vi "R30_1-FPGA.vi"() -> ()   [LabVIEW 2016]
uses:
  control vi/controls/Glassman Control.ctl
  control vi/controls/Faraday Cup Readback.ctl
  control vi/controls/Aperture Readback.ctl
  <vilib>/LabVIEW Targets/FPGA/cRIO/shared/nicrio_ModuleControls/nicrio_cRIO-9871_BaudRateEnum.ctl
  <vilib>/LabVIEW Targets/FPGA/cRIO/shared/nicrio_ModuleControls/nicrio_cRIO-9871_ParityEnum.ctl
  <vilib>/LabVIEW Targets/FPGA/cRIO/shared/nicrio_ModuleControls/nicrio_cRIO-9871_StopBitsEnum.ctl
  <vilib>/LabVIEW Targets/FPGA/cRIO/shared/nicrio_ModuleControls/nicrio_cRIO-9871_DataBitsEnum.ctl
  <vilib>/Platform/TimedLoop/XDataNode/timing_clust.ctl
  <vilib>/Platform/TimedLoop/XDataNode/nitl_modes.ctl
  <vilib>/Platform/TimedLoop/XDataNode/wakeup.ctl
  <vilib>/rvi/FXPMathLib/basic elements/FxpIntAccumulator/subVIs/nifxpmath_IntAccumulator_SimConfig.ctl
  <vilib>/rvi/Emulation/niFpgaGetClockAttributes.vi
  <vilib>/rvi/Emulation/niFpgaSctlEmulationGetInTimedLoop.vi
  <vilib>/rvi/Emulation/niFpgaEmulationReportErrorSimple.vi
  <vilib>/rvi/eio/common/nirviEmuTemplateMethod_errors.vi
  <vilib>/rvi/Analysis/common/codeGenErrors/XNode/niFpgaXNodeCodeGenErrorHandle.vi
  <vilib>/rvi/Emulation/niFpgaCriticalErrorInLSC.vi
  <vilib>/rvi/FXPMathLib/basic elements/FxpIntAccumulator/simVIs/DllFxpIntAccumulator_sub.vi
  <vilib>/rvi/eio/common/nirviEmuTemplatePropertySet_errors.vi
  <vilib>/eio/EIONode/EIONode.xnode
  <vilib>/rvi/Analysis/measure/dc-rms/XNode/niFpgaDC-RMS.xnode
  <vilib>/Platform/TimedLoop/XDataNode/XDataNode.xnode
  <vilib>/rvi/FXPMathLib/basic elements/FxpIntAccumulator/XNode/nifxpmath_IntAccumulator.xnode
  <vilib>/rvi/FXPMathLib/FxpMul/XNode/nifxpmath_Multiplier.xnode
  <vilib>/eio/EIOPropertyNode/EIOPropertyNode.xnode
  <vilib>/eio/EIOMethodNode/EIOMethodNode.xnode
  <vilib>/Platform/TimedLoop/XDataNode/XDNodeRunTimeDep.lvlib
  <vilib>/rvi/FXPMathLib/sim/FxpSim.dll
  <vilib>/rvi/eio/common/nirviEmuTemplatePropertyGet_errors.vi
  <vilib>/rvi/eio/common/nirviEmuTemplatePropertyGet_noerrors.vi
  <vilib>/rvi/eio/common/nirviEmuTemplatePropertySet_noerrors.vi
panel:
  out "ESA V read":fxp<+/-,26,5>
  out "ESA I read":fxp<+/-,26,5>
  out "X+ Steerer V read":fxp<+/-,26,5>
  out "X+ Steerer I read":fxp<+/-,26,5>
  out "X- Steerer V read":fxp<+/-,26,5>
  out "X- Steerer I read":fxp<+/-,26,5>
  out "Y+ Steerer V read":fxp<+/-,26,5>
  out "Y+ Steerer I read":fxp<+/-,26,5>
  out "Y- Steerer V read":fxp<+/-,26,5>
  out "Y- Steerer I read":fxp<+/-,26,5>
  out "Mag Steerer V read":fxp<+/-,26,5>
  out "Mag Steerer I read":fxp<+/-,26,5>
  out "HV readback loop error":errorcluster
  out "Quad B I read":fxp<+/-,26,5>
  out "Quad A I read":fxp<+/-,26,5>
  in  "RT error":bool
  out "Switch Magnet Aperture Position":T1
  out "Detector Aperture Position":T1
  out "Detector FC Position":T2
  out "Switch Magnet FC Position":T2
  out "Actuator loop error":errorcluster
  in  "Y- Steerer V set":T3
  in  "Y+ Steerer V set":T3
  in  "X- Steerer V set":T3
  in  "X+ Steerer V set":T3
  in  "Quad B set":fxp<+/-,20,5>
  in  "Quad A set":fxp<+/-,20,5>
  in  "ESA Voltage set":fxp<+/-,20,5>
  out "HV control loop error":errorcluster
  out "Cryo Readback error":errorcluster
  out "Vacuum Gauge 1 error":errorcluster
  out "Vacuum Gauge 2 error":errorcluster
  out "Vacuum Gauge 3 error":errorcluster
  out "Switch Image Ion Gauge 1":u8[](array[numeric])
  out "Switch Image Convectron 1":u8[](array[numeric])
  out "Time since repurge":u8[](array[numeric])
  out "1st stage temp":u8[](array[numeric])
  out "2nd stage temp":u8[](array[numeric])
  out "Cryo On-time":u8[](array[numeric])
  out "Cryo Status":u8[](array[numeric])
  out "R30 ESA Convectron  1":u8[](array[numeric])
  out "R30 ESA Ion gauge 1":u8[](array[numeric])
  out "R30 Detector Convectron  1":u8[](array[numeric])
  out "R30 Detector Ion gauge 1":u8[](array[numeric])
  in  "Mag Steerer I-program":fxp<+/-,20,5> format="%.17g"
  in  "Switch magnet Aperture Actuator":bool
  in  "Detector Aperture Actuator":bool
  in  "Detector FC Actuator":bool
  in  "Switch magnet FC Actuator":bool
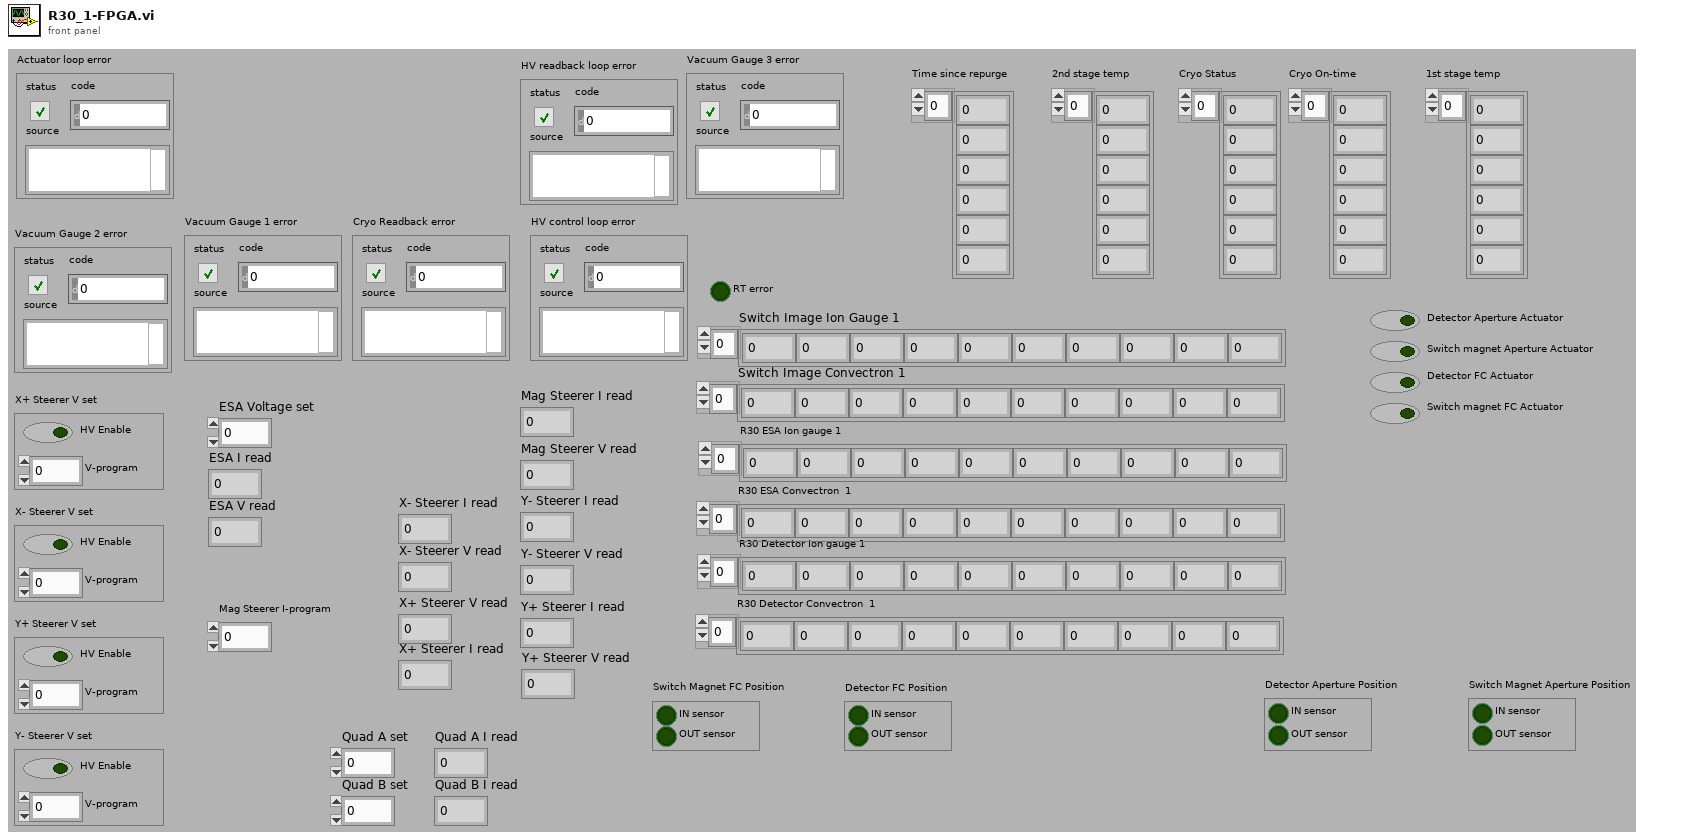
[diagram p1: front panel]
types:
  T1 = typedef "Aperture Readback.ctl" = cluster{"IN sensor":bool, "OUT sensor":bool}
  T2 = typedef "Faraday Cup Readback.ctl" = cluster{"IN sensor":bool, "OUT sensor":bool}
  T3 = typedef "Glassman Control.ctl" = cluster{"V-program":fxp<+/-,16,5>, "HV Enable":bool}
  T4 = typedef "nicrio_cRIO-9871_StopBitsEnum.ctl" = enum8{"1", "1.5", "2"}
  T5 = typedef "nicrio_cRIO-9871_ParityEnum.ctl" = enum8{"None", "Odd", "Even", "Mark", "Space"}
  T6 = typedef "nicrio_cRIO-9871_DataBitsEnum.ctl" = enum8{"5", "6", "7", "8"}
  T7 = typedef "nicrio_cRIO-9871_BaudRateEnum.ctl" = enum16{"75 bps", "110 bps", "134 bps", "150 bps", "300 bps", "600 bps", "1200 bps", "1800 bps", "2400 bps", "4800 bps", "7200 bps", "9600 bps", "14.4 kbps", "19.2 kbps", "28.8 kbps", "38.4 kbps", "57.6 kbps", "115.2 kbps", "230.4 kbps", "460.8 kbps", "921.6 kbps"}
  T8 = typedef "XDNodeRunTimeDep.lvlib/timing_clust.ctl" = cluster{"Expected End [f-1]":u64, "Actual End [f-1]":u64, "Finished Late? [f-1]":bool, "Expected End [i-1]":u64, "Actual End [i-1]":u64, "Finished Late? [i-1]":bool, "Expected Start [i]":u64, "Actual Start [i]":u64, "Expected Start [f]":u64, "Actual Start [f]":u64, "Source Name":string, "Structure Name":string, "Period":i64, "Deadline":i64, "Offset":i64, "Start":i64, "Priority":i32, "Timeout":i32, "Mode":T9, "Wakeup Reason":T10, "Error":errorcluster, "Source Type":string, "Secondary Source Type":string, "Global End Time":u64, "Global Start Time":u64, "Frame Duration":u64, "Iteration Duration":u64, "Assigned CPU":i32, "I/O Scan Engine Mode":u32}
  T9 = typedef "XDNodeRunTimeDep.lvlib/nitl_modes.ctl" = enum32{"No Change", "Process missed periods, maintain original phase", "Discard missed periods, maintain original phase", "Process missed periods, ignore original phase", "Discard missed periods, ignore original phase"}
  T10 = typedef "XDNodeRunTimeDep.lvlib/wakeup.ctl" = enum32{"Normal", "Aborted", "Asynchronous wakeup", "Timing source error", "Timed loop error", "Timeout"}
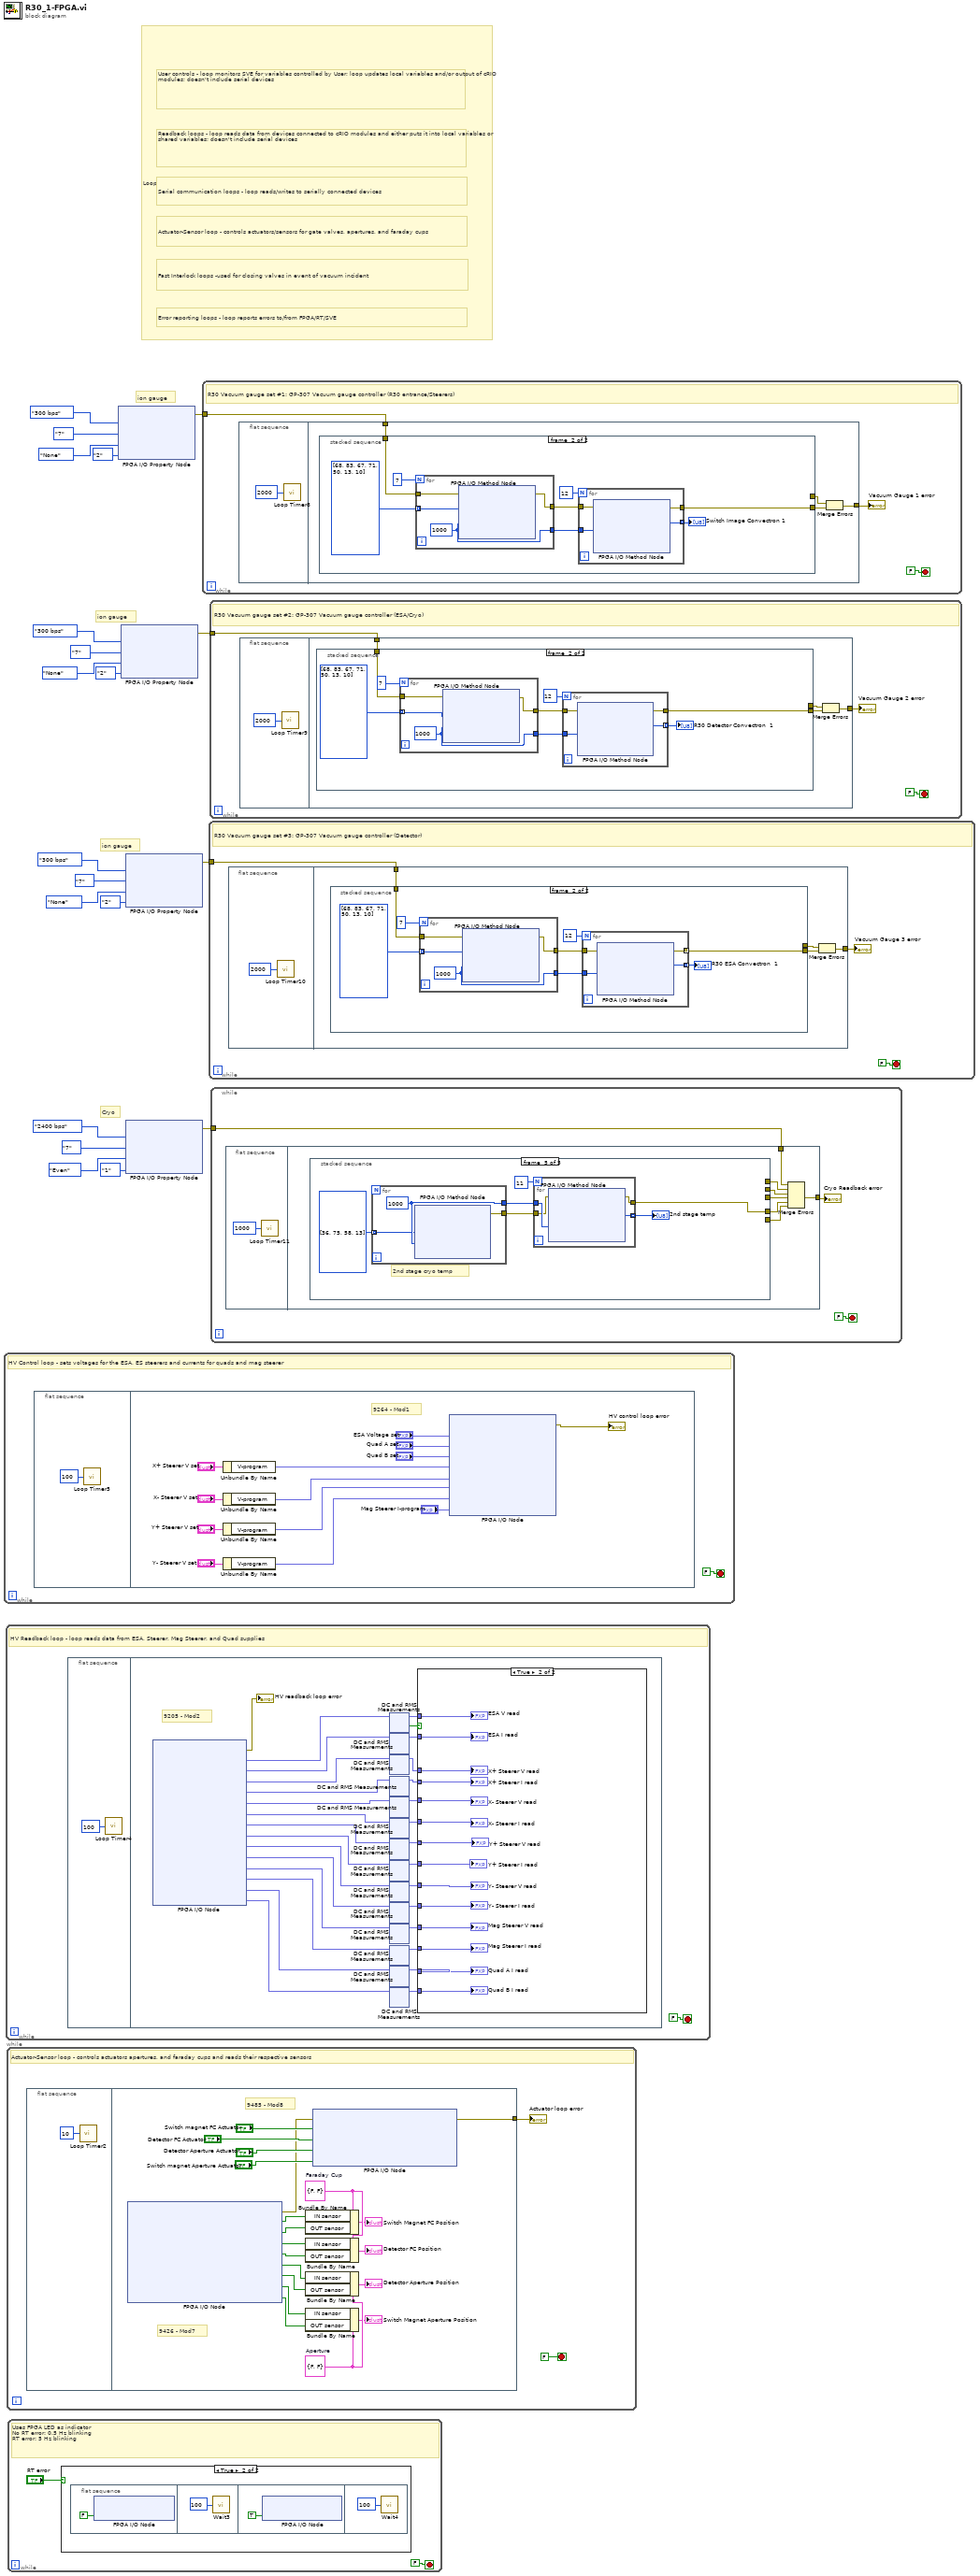
[diagram p0: block diagram]
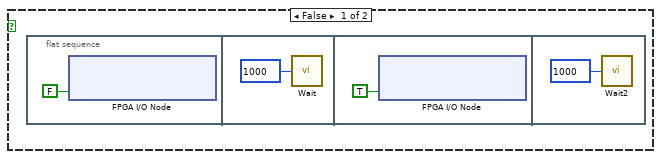
[diagram p2: hidden frame]
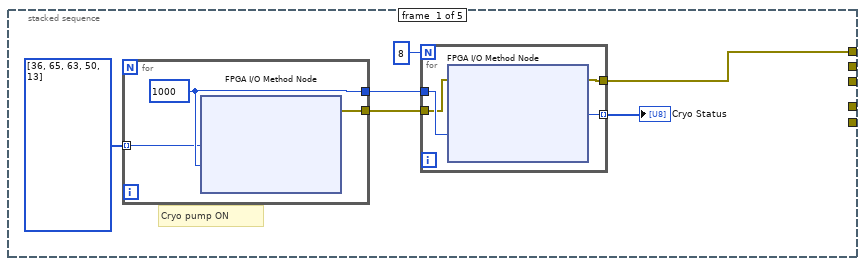
[diagram p3: hidden frame]
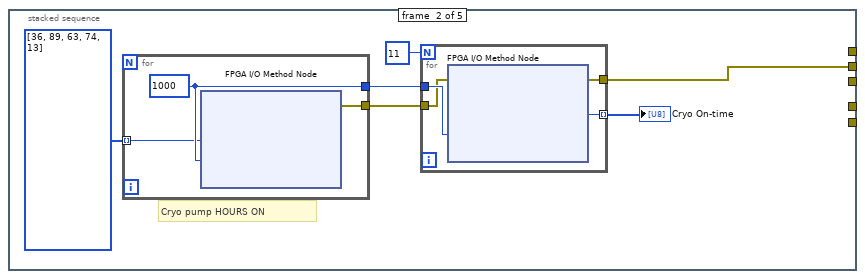
[diagram p4: hidden frame]
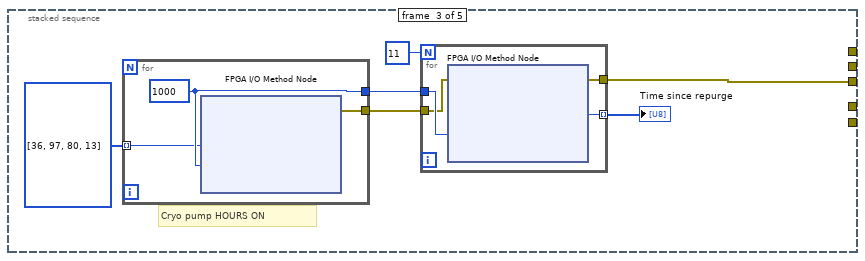
[diagram p5: hidden frame]
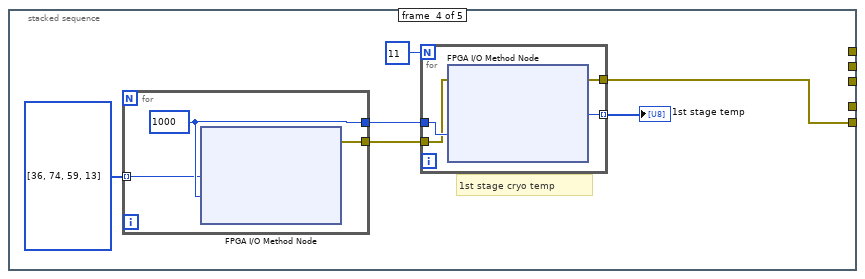
[diagram p6: hidden frame]
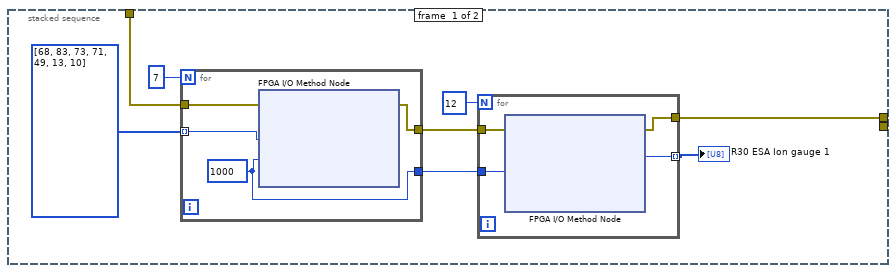
[diagram p7: hidden frame]
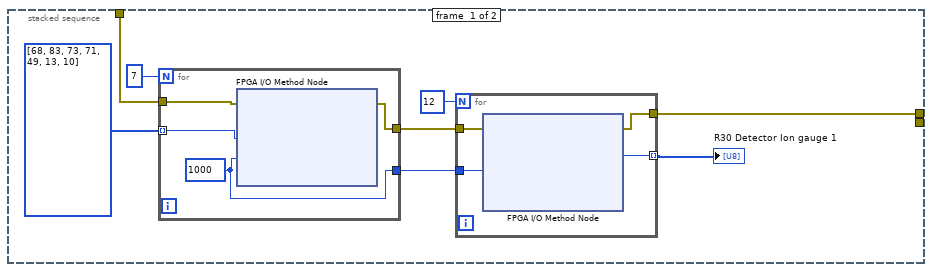
[diagram p8: hidden frame]
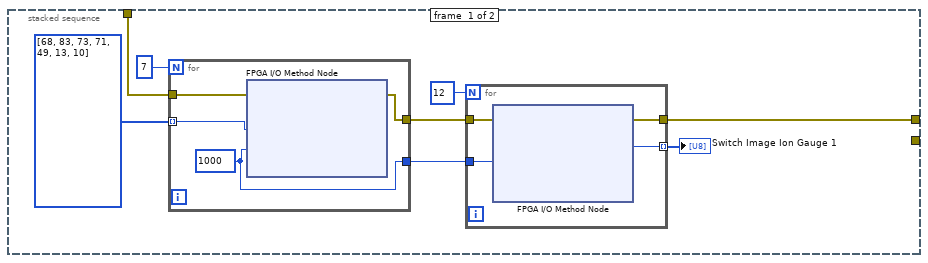
[diagram p9: hidden frame]
diagram:
  # "Actuator-Sensor loop - controls actuators/sensors for gate valves, apertures, and faraday cups"
  # "Fast Interlock loops -used for closing valves in event of vacuum incident"
  # "Error reporting loops - loop reports errors to/from FPGA/RT/SVE"
  # "Serial communication loops - loop reads/writes to serially connected devices"
  # "Readback loops - loop reads data from devices connected to cRIO modules and either puts it into local variables or shared variables; doesn't include serial devices"
  # "User controls - loop monitors SVE for variables controlled by User; loop updates local variables and/or output of cRIO modules; doesn't include serial devices"
  # "Loop legend - loops are color coded by responsibility"
  # "Cryo"
  # "ion gauge"
  # "ion gauge"
  # "ion gauge"
  n1 = while {
    stop <- FALSE stop-if-true
    # "HV Control loop - sets voltages for the ESA, ES steerers and currents for quads and mag steerer"
    n2 = flat-sequence {
      frame #0 {
        n3 = call "Loop Timer5"("Count(mSec)"=u32 100) -> ()  [unwired: 1 out]
      }
      frame #1 {
        # "9264 - Mod1"
        n4 = Unbundle By Name("X+ Steerer V set") -> ("V-program"=w26:fxp<+/-,16,5>)
        n5 = Unbundle By Name("X- Steerer V set") -> ("V-program"=w25:fxp<+/-,16,5>)
        n6 = Unbundle By Name("Y+ Steerer V set") -> ("V-program"=w24:fxp<+/-,16,5>)
        n7 = Unbundle By Name("Y- Steerer V set") -> ("V-program"=w23:fxp<+/-,16,5>)
        n8 = xnode "FPGA I/O Node"("ESA Voltage set"="ESA Voltage set", "Quad A set"="Quad A set", "Quad B set"="Quad B set", "X+ Steerer V set"=w26, "X- Steerer V set"=w25, "Y+ Steerer V set"=w24, "Y- Steerer V set"=w23, "Mag Steerer I-program"="Mag Steerer I-program") -> ("error out"=→"HV control loop error":errorcluster)  [unwired: 9 in, 8 out]
      }
    }
  }
  n9 = while {
    stop <- FALSE stop-if-true
    # "HV Readback loop - loop reads data from ESA, Steerer, Mag Steerer, and Quad supplies"
    n10 = flat-sequence {
      frame #0 {
        n11 = call "Loop Timer4"("Count(mSec)"=u32 100 ("Count(Ticks)")) -> ()  [unwired: 1 out]
      }
      frame #1 {
        # "9205 - Mod2"
        n12 = xnode "FPGA I/O Node"() -> ("error out"=→"HV readback loop error":errorcluster, "ESA V read"=w58:fxp<+/-,26,5>, "ESA I read"=w57:fxp<+/-,26,5>, "X+ Steerer V read"=w56:fxp<+/-,26,5>, "X+ Steerer I read"=w55:fxp<+/-,26,5>, "X- Steerer V read"=w54:fxp<+/-,26,5>, "X- Steerer I read"=w53:fxp<+/-,26,5>, "Y+ Steerer V read"=w52:fxp<+/-,26,5>, "Y+ Steerer I read"=w51:fxp<+/-,26,5>, "Y- Steerer V read"=w46:fxp<+/-,26,5>, "Y- Steerer I read"=w45:fxp<+/-,26,5>, "Mag Steerer V read"=w44:fxp<+/-,26,5>, "Mag Steerer I read"=w43:fxp<+/-,26,5>, "Quad A I read"=w42:fxp<+/-,26,5>, "Quad B I read"=w41:fxp<+/-,26,5>)  [unwired: 15 in, 14 out]
        n13 = xnode "DC and RMS Measurements"("input data"=w58) -> ("DC"=w66:fxp<+/-,26,5>, "output valid"=w67:bool)  [unwired: 1 in]
        n14 = xnode "DC and RMS Measurements"("input data"=w57) -> ("DC"=w65:fxp<+/-,26,5>)  [unwired: 1 in, 1 out]
        n15 = xnode "DC and RMS Measurements"("input data"=w56) -> ("DC"=w64:fxp<+/-,26,5>)  [unwired: 1 in, 1 out]
        n16 = xnode "DC and RMS Measurements"("input data"=w55) -> ("DC"=w63:fxp<+/-,26,5>)  [unwired: 1 in, 1 out]
        n17 = xnode "DC and RMS Measurements"("input data"=w54) -> ("DC"=w62:fxp<+/-,26,5>)  [unwired: 1 in, 1 out]
        n18 = xnode "DC and RMS Measurements"("input data"=w53) -> ("DC"=w61:fxp<+/-,26,5>)  [unwired: 1 in, 1 out]
        n19 = xnode "DC and RMS Measurements"("input data"=w52) -> ("DC"=w60:fxp<+/-,26,5>)  [unwired: 1 in, 1 out]
        n20 = xnode "DC and RMS Measurements"("input data"=w51) -> ("DC"=w59:fxp<+/-,26,5>)  [unwired: 1 in, 1 out]
        n21 = xnode "DC and RMS Measurements"("input data"=w46) -> ("DC"=w50:fxp<+/-,26,5>)  [unwired: 1 in, 1 out]
        n22 = xnode "DC and RMS Measurements"("input data"=w45) -> ("DC"=w49:fxp<+/-,26,5>)  [unwired: 1 in, 1 out]
        n23 = xnode "DC and RMS Measurements"("input data"=w44) -> ("DC"=w48:fxp<+/-,26,5>)  [unwired: 1 in, 1 out]
        n24 = xnode "DC and RMS Measurements"("input data"=w43) -> ("DC"=w47:fxp<+/-,26,5>)  [unwired: 1 in, 1 out]
        n25 = xnode "DC and RMS Measurements"("input data"=w42) -> ("DC"=w40:fxp<+/-,26,5>)  [unwired: 1 in, 1 out]
        n26 = xnode "DC and RMS Measurements"("input data"=w41) -> ("DC"=w39:fxp<+/-,26,5>)  [unwired: 1 in, 1 out]
        n27 = case shown="True" w67 {
          tunnel: w66 -> [_ w721]
          tunnel: w65 -> [_ w720]
          tunnel: w64 -> [_ w719]
          tunnel: w63 -> [_ w718]
          tunnel: w62 -> [_ w717]
          tunnel: w61 -> [_ w716]
          tunnel: w60 -> [_ w715]
          tunnel: w59 -> [_ w714]
          tunnel: w50 -> [_ w713]
          tunnel: w49 -> [_ w712]
          tunnel: w48 -> [_ w711]
          tunnel: w47 -> [_ w710]
          tunnel: w40 -> [_ w709]
          tunnel: w39 -> [_ w708]
          frame False {
          }
          frame True {
            "Quad A I read" <- w709
            "Quad B I read" <- w708
            "Mag Steerer I read" <- w710
            "Mag Steerer V read" <- w711
            "Y- Steerer I read" <- w712
            "Y- Steerer V read" <- w713
            "Y+ Steerer I read" <- w714
            "Y+ Steerer V read" <- w715
            "X- Steerer I read" <- w716
            "X- Steerer V read" <- w717
            "X+ Steerer I read" <- w718
            "X+ Steerer V read" <- w719
            "ESA I read" <- w720
            "ESA V read" <- w721
          }
        }
      }
    }
  }
  n28 = while {
    stop <- FALSE stop-if-true
    # "Actuator-Sensor loop - controls actuators apertures, and faraday cups and reads their respective sensors"
    n29 = flat-sequence {
      tunnel: [w1222] -> w1202
      frame #0 {
        n30 = call "Loop Timer2"("Count(uSec)"=u32 10) -> ()  [unwired: 1 out]
      }
      frame #1 {
        w1211 = T1 {"IN sensor"=FALSE, "OUT sensor"=FALSE}  # Aperture
        w1214 = T2 {"IN sensor"=FALSE, "OUT sensor"=FALSE}  # Faraday Cup
        # "9485 - Mod8"
        # "9426 - Mod7"
        n31 = xnode "FPGA I/O Node"() -> ("error out"=w1219:errorcluster, "Switch Magnet FC IN sensor"=w1218:bool, "Switch Magnet FC OUT sensor"=w1217:bool, "Detector FC IN sensor"=w1216:bool, "Detector FC OUT sensor"=w1215:bool, "Detector Aperture IN sensor"=w1207:bool, "Detector Aperture OUT sensor"=w1208:bool, "Switch Magnet Aperture IN sensor"=w1209:bool, "Switch Magnet Aperture OUT sensor"=w1210:bool)  [unwired: 9 in, 8 out]
        n32 = Bundle By Name(cluster=w1214, "IN sensor"=w1218, "OUT sensor"=w1217) -> (→"Switch Magnet FC Position":T2)
        n33 = Bundle By Name(cluster=w1214, "IN sensor"=w1216, "OUT sensor"=w1215) -> (→"Detector FC Position":T2)
        n34 = Bundle By Name(cluster=w1211, "IN sensor"=w1207, "OUT sensor"=w1208) -> (→"Detector Aperture Position":T1)
        n35 = Bundle By Name(cluster=w1211, "IN sensor"=w1209, "OUT sensor"=w1210) -> (→"Switch Magnet Aperture Position":T1)
        n36 = xnode "FPGA I/O Node"("error in"=w1219, "Switch Magnet FC Actuator"="Switch magnet FC Actuator", "Detector FC Actuator"="Detector FC Actuator", "Detector Aperture Actuator"="Detector Aperture Actuator", "Switch Magnet Aperture Actuator"="Switch magnet Aperture Actuator") -> ("error out"=w1222:errorcluster)  [unwired: 4 in, 4 out]
      }
    }
    "Actuator loop error" <- w1202
  }
  n37 = while {
    stop <- FALSE stop-if-true
    # "Uses FPGA LED as indicator\nNo RT error: 0.5 Hz blinking\nRT error: 5 Hz blinking"
    n38 = case shown="True" "RT error" {
      frame False {
        n39 = flat-sequence {
          frame #0 {
            n40 = xnode "FPGA I/O Node"("USER FPGA LED"=FALSE ("FPGA LED")) -> ()  [unwired: 1 in, 1 out]
          }
          frame #1 {
            n41 = call "Wait"("Count(mSec)"=u16 1000) -> ()  [unwired: 1 out]
          }
          frame #2 {
            n42 = xnode "FPGA I/O Node"("USER FPGA LED"=TRUE ("FPGA LED")) -> ()  [unwired: 1 in, 1 out]
          }
          frame #3 {
            n43 = call "Wait2"("Count(mSec)"=u16 1000) -> ()  [unwired: 1 out]
          }
        }
      }
      frame True {
        n44 = flat-sequence {
          frame #0 {
            n45 = xnode "FPGA I/O Node"("USER FPGA LED"=FALSE ("FPGA LED")) -> ()  [unwired: 1 in, 1 out]
          }
          frame #1 {
            n46 = call "Wait3"("Count(mSec)"=u16 100) -> ()  [unwired: 1 out]
          }
          frame #2 {
            n47 = xnode "FPGA I/O Node"("USER FPGA LED"=TRUE ("FPGA LED")) -> ()  [unwired: 1 in, 1 out]
          }
          frame #3 {
            n48 = call "Wait4"("Count(mSec)"=u16 100) -> ()  [unwired: 1 out]
          }
        }
      }
    }
  }
  n49 = xnode "FPGA I/O Property Node"("Baud Rate"=nicrio_cRIO-9871_BaudRateEnum."300 bps", "Data Bits"=nicrio_cRIO-9871_DataBitsEnum."7", "Parity"=nicrio_cRIO-9871_ParityEnum."None", "Stop Bits"=nicrio_cRIO-9871_StopBitsEnum."2") -> ("error out"=w4:errorcluster)  [unwired: 2 in, 1 out]
  n50 = xnode "FPGA I/O Property Node"("Baud Rate"=nicrio_cRIO-9871_BaudRateEnum."300 bps", "Data Bits"=nicrio_cRIO-9871_DataBitsEnum."7", "Parity"=nicrio_cRIO-9871_ParityEnum."None", "Stop Bits"=nicrio_cRIO-9871_StopBitsEnum."2") -> ("error out"=w3:errorcluster)  [unwired: 2 in, 1 out]
  n51 = xnode "FPGA I/O Property Node"("Baud Rate"=nicrio_cRIO-9871_BaudRateEnum."300 bps", "Data Bits"=nicrio_cRIO-9871_DataBitsEnum."7", "Parity"=nicrio_cRIO-9871_ParityEnum."None", "Stop Bits"=nicrio_cRIO-9871_StopBitsEnum."2") -> ("error out"=w2:errorcluster)  [unwired: 2 in, 1 out]
  n52 = xnode "FPGA I/O Property Node"("Baud Rate"=nicrio_cRIO-9871_BaudRateEnum."2400 bps", "Data Bits"=nicrio_cRIO-9871_DataBitsEnum."7", "Parity"=nicrio_cRIO-9871_ParityEnum."Even", "Stop Bits"=nicrio_cRIO-9871_StopBitsEnum."1") -> ("error out"=w1:errorcluster)  [unwired: 2 in, 1 out]
  n53 = while {
    tunnel: w4 -> [w1236]
    stop <- FALSE stop-if-true
    # "R30 Vacuum gauge set #1: GP-307 Vacuum gauge controller (R30 entrance/Steerers)"
    n54 = flat-sequence {
      tunnel: w1236 -> [w1242]
      tunnel: [w1239] -> w1235
      frame #0 {
        n55 = call "Loop Timer8"("Count(mSec)"=u32 2000 ("Count(Ticks)")) -> ()  [unwired: 1 out]
      }
      frame #1 {
        n56 = stacked-sequence {
          tunnel: w1242 -> [w1245 w1261]
          tunnel: [_ w1259] -> w1241
          tunnel: [w1243 _] -> w1240
          frame #0 {
            n57 = for {
              N: 7 -> [_]
              tunnel: [w1257] -> w1250
              tunnel: u8[] [68, 83, 73, 71, 49, 13, 10] ("unsigned byte array") -> [w1258] mode=indexing
              tunnel: w1245 -> [w1256]
              tunnel: [w1255] -> w1244
              w1257 = 1000 ("Timeout (ms)")
              n58 = xnode "FPGA I/O Method Node"("error in"=w1256, "Data"=w1258, "Timeout (ms)"=w1257) -> ("error out"=w1255:errorcluster)  [unwired: 1 in, 2 out]
            }
            n59 = for {
              N: 12 -> [_]
              tunnel: w1250 -> [w1254]
              tunnel: [w1253] -> w1246 mode=indexing
              tunnel: w1244 -> [w1252]
              tunnel: [w1251] -> w1243
              n60 = xnode "FPGA I/O Method Node"("error in"=w1252, "Timeout (ms)"=w1254) -> ("error out"=w1251:errorcluster, "Data"=w1253:u8)  [unwired: 1 in, 2 out]
            }
            "Switch Image Ion Gauge 1" <- w1246
          }
          frame #1 {
            n61 = for {
              N: 7 -> [_]
              tunnel: [w1273] -> w1266
              tunnel: u8[] [68, 83, 67, 71, 50, 13, 10] ("unsigned byte array") -> [w1274] mode=indexing
              tunnel: w1261 -> [w1272]
              tunnel: [w1271] -> w1260
              w1273 = 1000 ("Timeout (ms)")
              n62 = xnode "FPGA I/O Method Node"("error in"=w1272, "Data"=w1274, "Timeout (ms)"=w1273) -> ("error out"=w1271:errorcluster)  [unwired: 1 in, 2 out]
            }
            n63 = for {
              N: 12 -> [_]
              tunnel: w1266 -> [w1270]
              tunnel: [w1269] -> w1262 mode=indexing
              tunnel: w1260 -> [w1268]
              tunnel: [w1267] -> w1259
              n64 = xnode "FPGA I/O Method Node"("error in"=w1268, "Timeout (ms)"=w1270) -> ("error out"=w1267:errorcluster, "Data"=w1269:u8)  [unwired: 1 in, 2 out]
            }
            "Switch Image Convectron 1" <- w1262
          }
        }
        n65 = Merge Errors(w1240, w1241) -> (w1239:errorcluster)
      }
    }
    "Vacuum Gauge 1 error" <- w1235
  }
  n66 = while {
    tunnel: w2 -> [w1276]
    stop <- FALSE stop-if-true
    # "R30 Vacuum gauge set #3: GP-307 Vacuum gauge controller (Detector)"
    n67 = flat-sequence {
      tunnel: w1276 -> [w1282]
      tunnel: [w1279] -> w1275
      frame #0 {
        n68 = call "Loop Timer10"("Count(mSec)"=u32 2000 ("Count(Ticks)")) -> ()  [unwired: 1 out]
      }
      frame #1 {
        n69 = stacked-sequence {
          tunnel: w1282 -> [w1285 w1301]
          tunnel: [_ w1299] -> w1281
          tunnel: [w1283 _] -> w1280
          frame #0 {
            n70 = for {
              N: 7 -> [_]
              tunnel: [w1297] -> w1290
              tunnel: u8[] [68, 83, 73, 71, 49, 13, 10] ("unsigned byte array") -> [w1298] mode=indexing
              tunnel: w1285 -> [w1296]
              tunnel: [w1295] -> w1284
              w1297 = 1000 ("Timeout (ms)")
              n71 = xnode "FPGA I/O Method Node"("error in"=w1296, "Data"=w1298, "Timeout (ms)"=w1297) -> ("error out"=w1295:errorcluster)  [unwired: 1 in, 2 out]
            }
            n72 = for {
              N: 12 -> [_]
              tunnel: w1290 -> [w1294]
              tunnel: [w1293] -> w1286 mode=indexing
              tunnel: w1284 -> [w1292]
              tunnel: [w1291] -> w1283
              n73 = xnode "FPGA I/O Method Node"("error in"=w1292, "Timeout (ms)"=w1294) -> ("error out"=w1291:errorcluster, "Data"=w1293:u8)  [unwired: 1 in, 2 out]
            }
            "R30 ESA Ion gauge 1" <- w1286
          }
          frame #1 {
            n74 = for {
              N: 7 -> [_]
              tunnel: [w1313] -> w1306
              tunnel: u8[] [68, 83, 67, 71, 50, 13, 10] ("unsigned byte array") -> [w1314] mode=indexing
              tunnel: w1301 -> [w1312]
              tunnel: [w1311] -> w1300
              w1313 = 1000 ("Timeout (ms)")
              n75 = xnode "FPGA I/O Method Node"("error in"=w1312, "Data"=w1314, "Timeout (ms)"=w1313) -> ("error out"=w1311:errorcluster)  [unwired: 1 in, 2 out]
            }
            n76 = for {
              N: 12 -> [_]
              tunnel: w1306 -> [w1310]
              tunnel: [w1309] -> w1302 mode=indexing
              tunnel: w1300 -> [w1308]
              tunnel: [w1307] -> w1299 mode=indexing
              n77 = xnode "FPGA I/O Method Node"("error in"=w1308, "Timeout (ms)"=w1310) -> ("error out"=w1307:errorcluster, "Data"=w1309:u8)  [unwired: 1 in, 2 out]
            }
            "R30 ESA Convectron  1" <- w1302
          }
        }
        n78 = Merge Errors(w1280, w1281) -> (w1279:errorcluster)
      }
    }
    "Vacuum Gauge 3 error" <- w1275
  }
  n79 = while {
    tunnel: w3 -> [w1316]
    stop <- FALSE stop-if-true
    # "R30 Vacuum gauge set #2: GP-307 Vacuum gauge controller (ESA/Cryo)"
    n80 = flat-sequence {
      tunnel: w1316 -> [w1322]
      tunnel: [w1319] -> w1315
      frame #0 {
        n81 = call "Loop Timer9"("Count(mSec)"=u32 2000 ("Count(Ticks)")) -> ()  [unwired: 1 out]
      }
      frame #1 {
        n82 = stacked-sequence {
          tunnel: w1322 -> [w1325 w1341]
          tunnel: [_ w1339] -> w1321
          tunnel: [w1323 _] -> w1320
          frame #0 {
            n83 = for {
              N: 7 -> [_]
              tunnel: [w1337] -> w1330
              tunnel: u8[] [68, 83, 73, 71, 49, 13, 10] ("unsigned byte array") -> [w1338] mode=indexing
              tunnel: w1325 -> [w1336]
              tunnel: [w1335] -> w1324
              w1337 = 1000 ("Timeout (ms)")
              n84 = xnode "FPGA I/O Method Node"("error in"=w1336, "Data"=w1338, "Timeout (ms)"=w1337) -> ("error out"=w1335:errorcluster)  [unwired: 1 in, 2 out]
            }
            n85 = for {
              N: 12 -> [_]
              tunnel: w1330 -> [w1334]
              tunnel: [w1333] -> w1326 mode=indexing
              tunnel: w1324 -> [w1332]
              tunnel: [w1331] -> w1323
              n86 = xnode "FPGA I/O Method Node"("error in"=w1332, "Timeout (ms)"=w1334) -> ("error out"=w1331:errorcluster, "Data"=w1333:u8)  [unwired: 1 in, 2 out]
            }
            "R30 Detector Ion gauge 1" <- w1326
          }
          frame #1 {
            n87 = for {
              N: 7 -> [_]
              tunnel: [w1353] -> w1346
              tunnel: u8[] [68, 83, 67, 71, 50, 13, 10] ("unsigned byte array") -> [w1354] mode=indexing
              tunnel: w1341 -> [w1352]
              tunnel: [w1351] -> w1340
              w1353 = 1000 ("Timeout (ms)")
              n88 = xnode "FPGA I/O Method Node"("error in"=w1352, "Data"=w1354, "Timeout (ms)"=w1353) -> ("error out"=w1351:errorcluster)  [unwired: 1 in, 2 out]
            }
            n89 = for {
              N: 12 -> [_]
              tunnel: w1346 -> [w1350]
              tunnel: [w1349] -> w1342 mode=indexing
              tunnel: w1340 -> [w1348]
              tunnel: [w1347] -> w1339
              n90 = xnode "FPGA I/O Method Node"("error in"=w1348, "Timeout (ms)"=w1350) -> ("error out"=w1347:errorcluster, "Data"=w1349:u8)  [unwired: 1 in, 2 out]
            }
            "R30 Detector Convectron  1" <- w1342
          }
        }
        n91 = Merge Errors(w1320, w1321) -> (w1319:errorcluster)
      }
    }
    "Vacuum Gauge 2 error" <- w1315
  }
  n92 = while {
    tunnel: w1 -> [w1355]
    stop <- FALSE stop-if-true
    n93 = flat-sequence {
      tunnel: [w1360] -> w1356
      tunnel: w1355 -> [w1359]
      frame #0 {
        n94 = call "Loop Timer11"("Count(mSec)"=u32 1000 ("Count(Ticks)")) -> ()  [unwired: 1 out]
      }
      frame #1 {
        n95 = stacked-sequence {
          tunnel: [w1367 _ _ _ _] -> w1365
          tunnel: [_ w1380 _ _ _] -> w1364
          tunnel: [_ _ w1392 _ _] -> w1363
          tunnel: [_ _ _ _ w1418] -> w1362
          tunnel: [_ _ _ w1405 _] -> w1361
          frame #0 {
            # "Cryo pump ON"
            n96 = for {
              tunnel: [w1378] -> w1371
              tunnel: u8[] [36, 65, 63, 50, 13] ("unsigned byte array") -> [w1377] mode=indexing
              tunnel: [w1376] -> w1366
              w1378 = 1000 ("Timeout (ms)")
              n97 = xnode "FPGA I/O Method Node"("Data"=w1377, "Timeout (ms)"=w1378) -> ("error out"=w1376:errorcluster)  [unwired: 2 in, 2 out]
            }
            n98 = for {
              N: 8 -> [_]
              tunnel: w1371 -> [w1375]
              tunnel: [w1374] -> w1368 mode=indexing
              tunnel: [w1373] -> w1367
              tunnel: w1366 -> [w1372]
              n99 = xnode "FPGA I/O Method Node"("error in"=w1372, "Timeout (ms)"=w1375) -> ("error out"=w1373:errorcluster, "Data"=w1374:u8)  [unwired: 1 in, 2 out]
            }
            "Cryo Status" <- w1368
          }
          frame #1 {
            # "Cryo pump HOURS ON"
            n100 = for {
              tunnel: [w1391] -> w1384
              tunnel: u8[] [36, 89, 63, 74, 13] ("unsigned byte array") -> [w1390] mode=indexing
              tunnel: [w1389] -> w1379
              w1391 = 1000 ("Timeout (ms)")
              n101 = xnode "FPGA I/O Method Node"("Data"=w1390, "Timeout (ms)"=w1391) -> ("error out"=w1389:errorcluster)  [unwired: 2 in, 2 out]
            }
            n102 = for {
              N: 11 -> [_]
              tunnel: w1384 -> [w1388]
              tunnel: [w1387] -> w1381 mode=indexing
              tunnel: [w1386] -> w1380
              tunnel: w1379 -> [w1385]
              n103 = xnode "FPGA I/O Method Node"("error in"=w1385, "Timeout (ms)"=w1388) -> ("error out"=w1386:errorcluster, "Data"=w1387:u8)  [unwired: 1 in, 2 out]
            }
            "Cryo On-time" <- w1381
          }
          frame #2 {
            # "Cryo pump HOURS ON"
            n104 = for {
              tunnel: [w1404] -> w1397
              tunnel: u8[] [36, 97, 80, 13] ("unsigned byte array") -> [w1403] mode=indexing
              tunnel: [w1402] -> w1393
              w1404 = 1000 ("Timeout (ms)")
              n105 = xnode "FPGA I/O Method Node"("Data"=w1403, "Timeout (ms)"=w1404) -> ("error out"=w1402:errorcluster)  [unwired: 2 in, 2 out]
            }
            n106 = for {
              N: 11 -> [_]
              tunnel: w1397 -> [w1401]
              tunnel: [w1400] -> w1394 mode=indexing
              tunnel: w1393 -> [w1399]
              tunnel: [w1398] -> w1392
              n107 = xnode "FPGA I/O Method Node"("error in"=w1399, "Timeout (ms)"=w1401) -> ("error out"=w1398:errorcluster, "Data"=w1400:u8)  [unwired: 1 in, 2 out]
            }
            "Time since repurge" <- w1394
          }
          frame #3 {
            # "1st stage cryo temp"
            n108 = for {
              tunnel: [w1417] -> w1410
              tunnel: u8[] [36, 74, 59, 13] ("unsigned byte array") -> [w1416] mode=indexing
              tunnel: [w1415] -> w1406
              w1417 = 1000 ("Timeout (ms)")
              n109 = xnode "FPGA I/O Method Node"("Data"=w1416, "Timeout (ms)"=w1417) -> ("error out"=w1415:errorcluster)  [unwired: 2 in, 2 out]
            }
            n110 = for {
              N: 11 -> [_]
              tunnel: w1410 -> [w1414]
              tunnel: [w1413] -> w1407 mode=indexing
              tunnel: w1406 -> [w1412]
              tunnel: [w1411] -> w1405
              n111 = xnode "FPGA I/O Method Node"("error in"=w1412, "Timeout (ms)"=w1414) -> ("error out"=w1411:errorcluster, "Data"=w1413:u8)  [unwired: 1 in, 2 out]
            }
            "1st stage temp" <- w1407
          }
          frame #4 {
            # "2nd stage cryo temp"
            n112 = for {
              tunnel: [w1430] -> w1423
              tunnel: u8[] [36, 75, 58, 13] ("unsigned byte array") -> [w1429] mode=indexing
              tunnel: [w1428] -> w1419
              w1430 = 1000 ("Timeout (ms)")
              n113 = xnode "FPGA I/O Method Node"("Data"=w1429, "Timeout (ms)"=w1430) -> ("error out"=w1428:errorcluster)  [unwired: 2 in, 2 out]
            }
            n114 = for {
              N: 11 -> [_]
              tunnel: w1423 -> [w1427]
              tunnel: [w1426] -> w1420 mode=indexing
              tunnel: w1419 -> [w1425]
              tunnel: [w1424] -> w1418
              n115 = xnode "FPGA I/O Method Node"("error in"=w1425, "Timeout (ms)"=w1427) -> ("error out"=w1424:errorcluster, "Data"=w1426:u8)  [unwired: 1 in, 2 out]
            }
            "2nd stage temp" <- w1420
          }
        }
        n116 = Merge Errors(w1359, w1365, w1364, w1363, w1362, w1361) -> (w1360:errorcluster)
      }
    }
    "Cryo Readback error" <- w1356
  }
